vi "USRP oneTx one Rx_USRP1.vi"() -> ()   [LabVIEW 2021]
uses:
  <vilib>/addons/Modulation/Analog/controls/Complex Data Waveform.ctl
  <vilib>/measure/maspectr.llb/Power Spectrum and PSD Export Mode.ctl
  system stop.vi
  <vilib>/measure/matone.llb/Extract Single Tone Information 1 Chan (CDB).vi
  <vilib>/measure/maspectr.llb/FFT Power Spectrum and PSD for 1 Chan (CDB).vi
  <instrlib>/niUSRP/niUSRP Fetch Rx Data (CDB Cluster).vi
  <instrlib>/niUSRP/niUSRP Write Tx Data (CDB Cluster).vi
  <vilib>/addons/Modulation/niAMT.lvlib
  <vilib>/measure/NI_MAPro.lvlib
panel:
  in  "Tab Control":T1(tab)
  in  "IQ rate Tx":dbl=100000.0 format="%#_6p"
  in  "carrier frequency Tx":dbl=100000.0 format="%#_6p"
  in  "Tx Gain":dbl format="%#_6f"
  in  "Tx IP":refnum<k15>
  out "coerced IQ rate Tx":dbl=100000.0 format="%#_6p"
  out "coerced carrier frequency Tx":dbl=100000.0 format="%#_6p"
  in  "Rx IP":refnum<k15>
  in  "Rx gain":dbl format="%#_6f"
  in  "Frequency":dbl format="%#_13g"
  in  "Duration":dbl format="%#_13g"
  out "coerced IQ rate Rx":dbl=100000.0 format="%#_6p"
  out "coerced carrier frequency Rx":dbl=100000.0 format="%#_6p"
  in  "number of samples":i64=100000
  out "Waveform Graph":dbl[](graph)
  out "Boolean":bool
  out "Received Waveform Graph":cluster{"f0":dbl, "df":dbl, "magnitude":dbl[]}(graph)
  out "detected frequency":dbl format="%.2p"
  out "detected Amplitude in dBm":dbl format="%.2p"
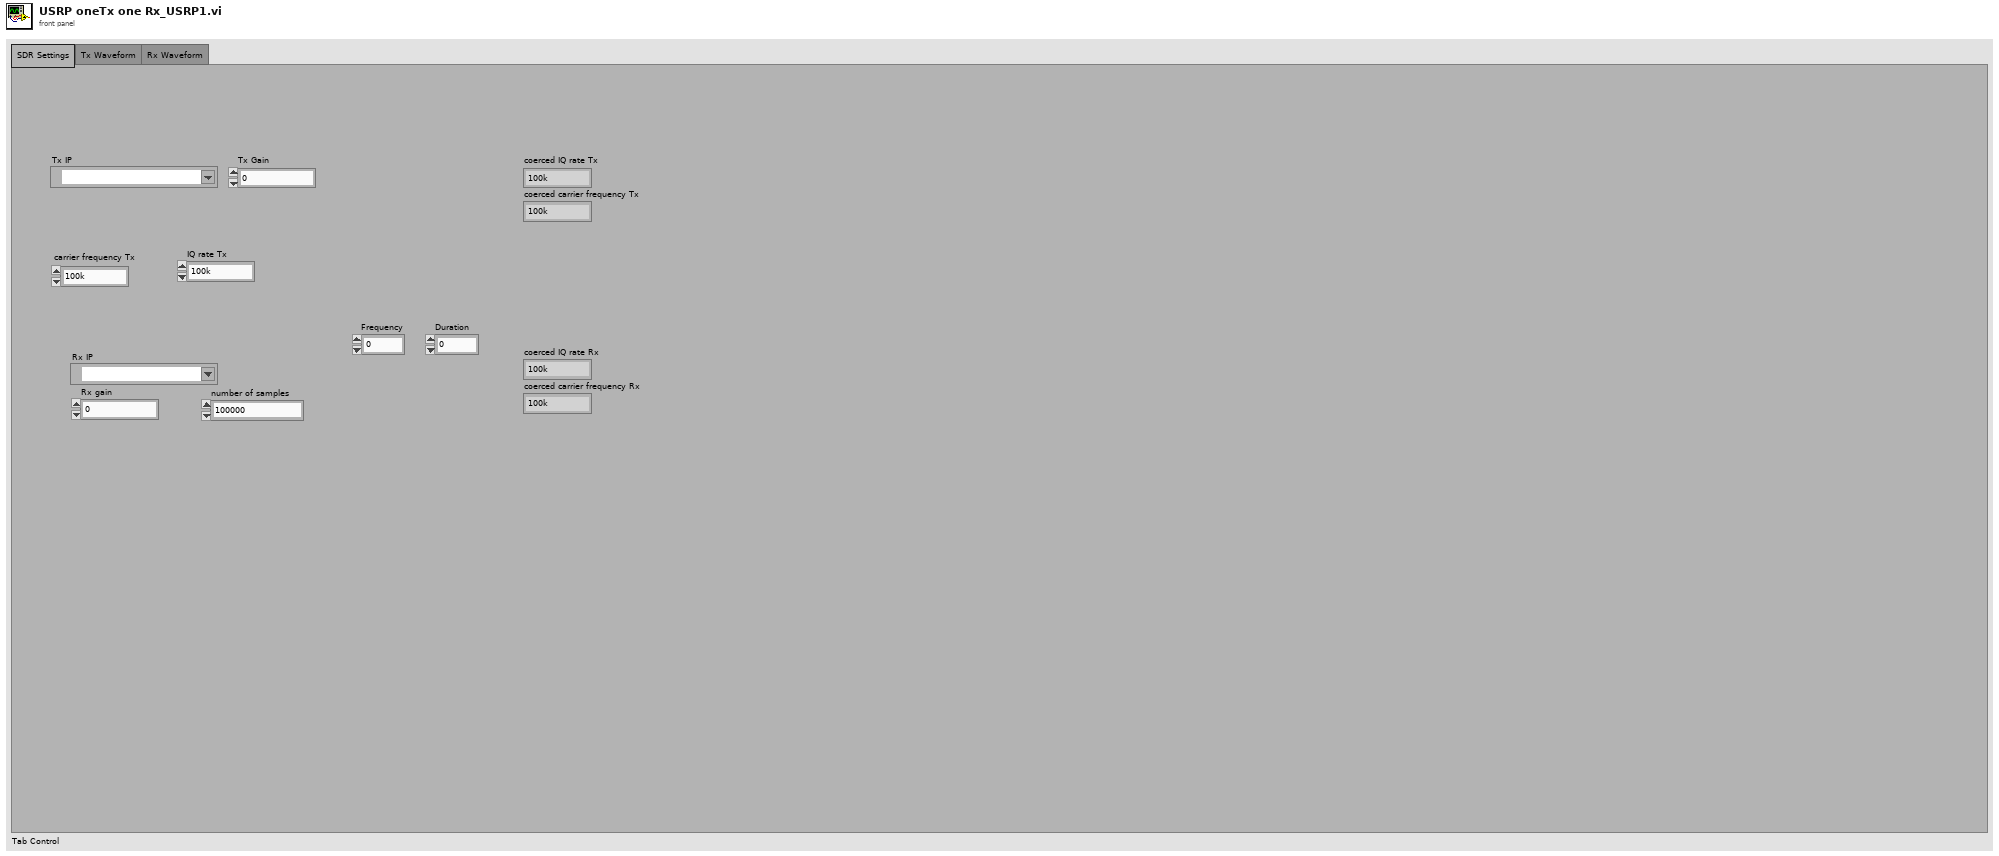
[diagram p1: front panel]
types:
  T1 = enum32{"SDR Settings", "Tx Waveform", "Rx Waveform"}
  T2 = typedef "niAMT.lvlib/Complex Data Waveform.ctl" = cluster{"t0":dbl, "dt":dbl, "Y":cdb[]}
  T3 = typedef "NI_MAPro.lvlib/Power Spectrum and PSD Export Mode.ctl" = u16
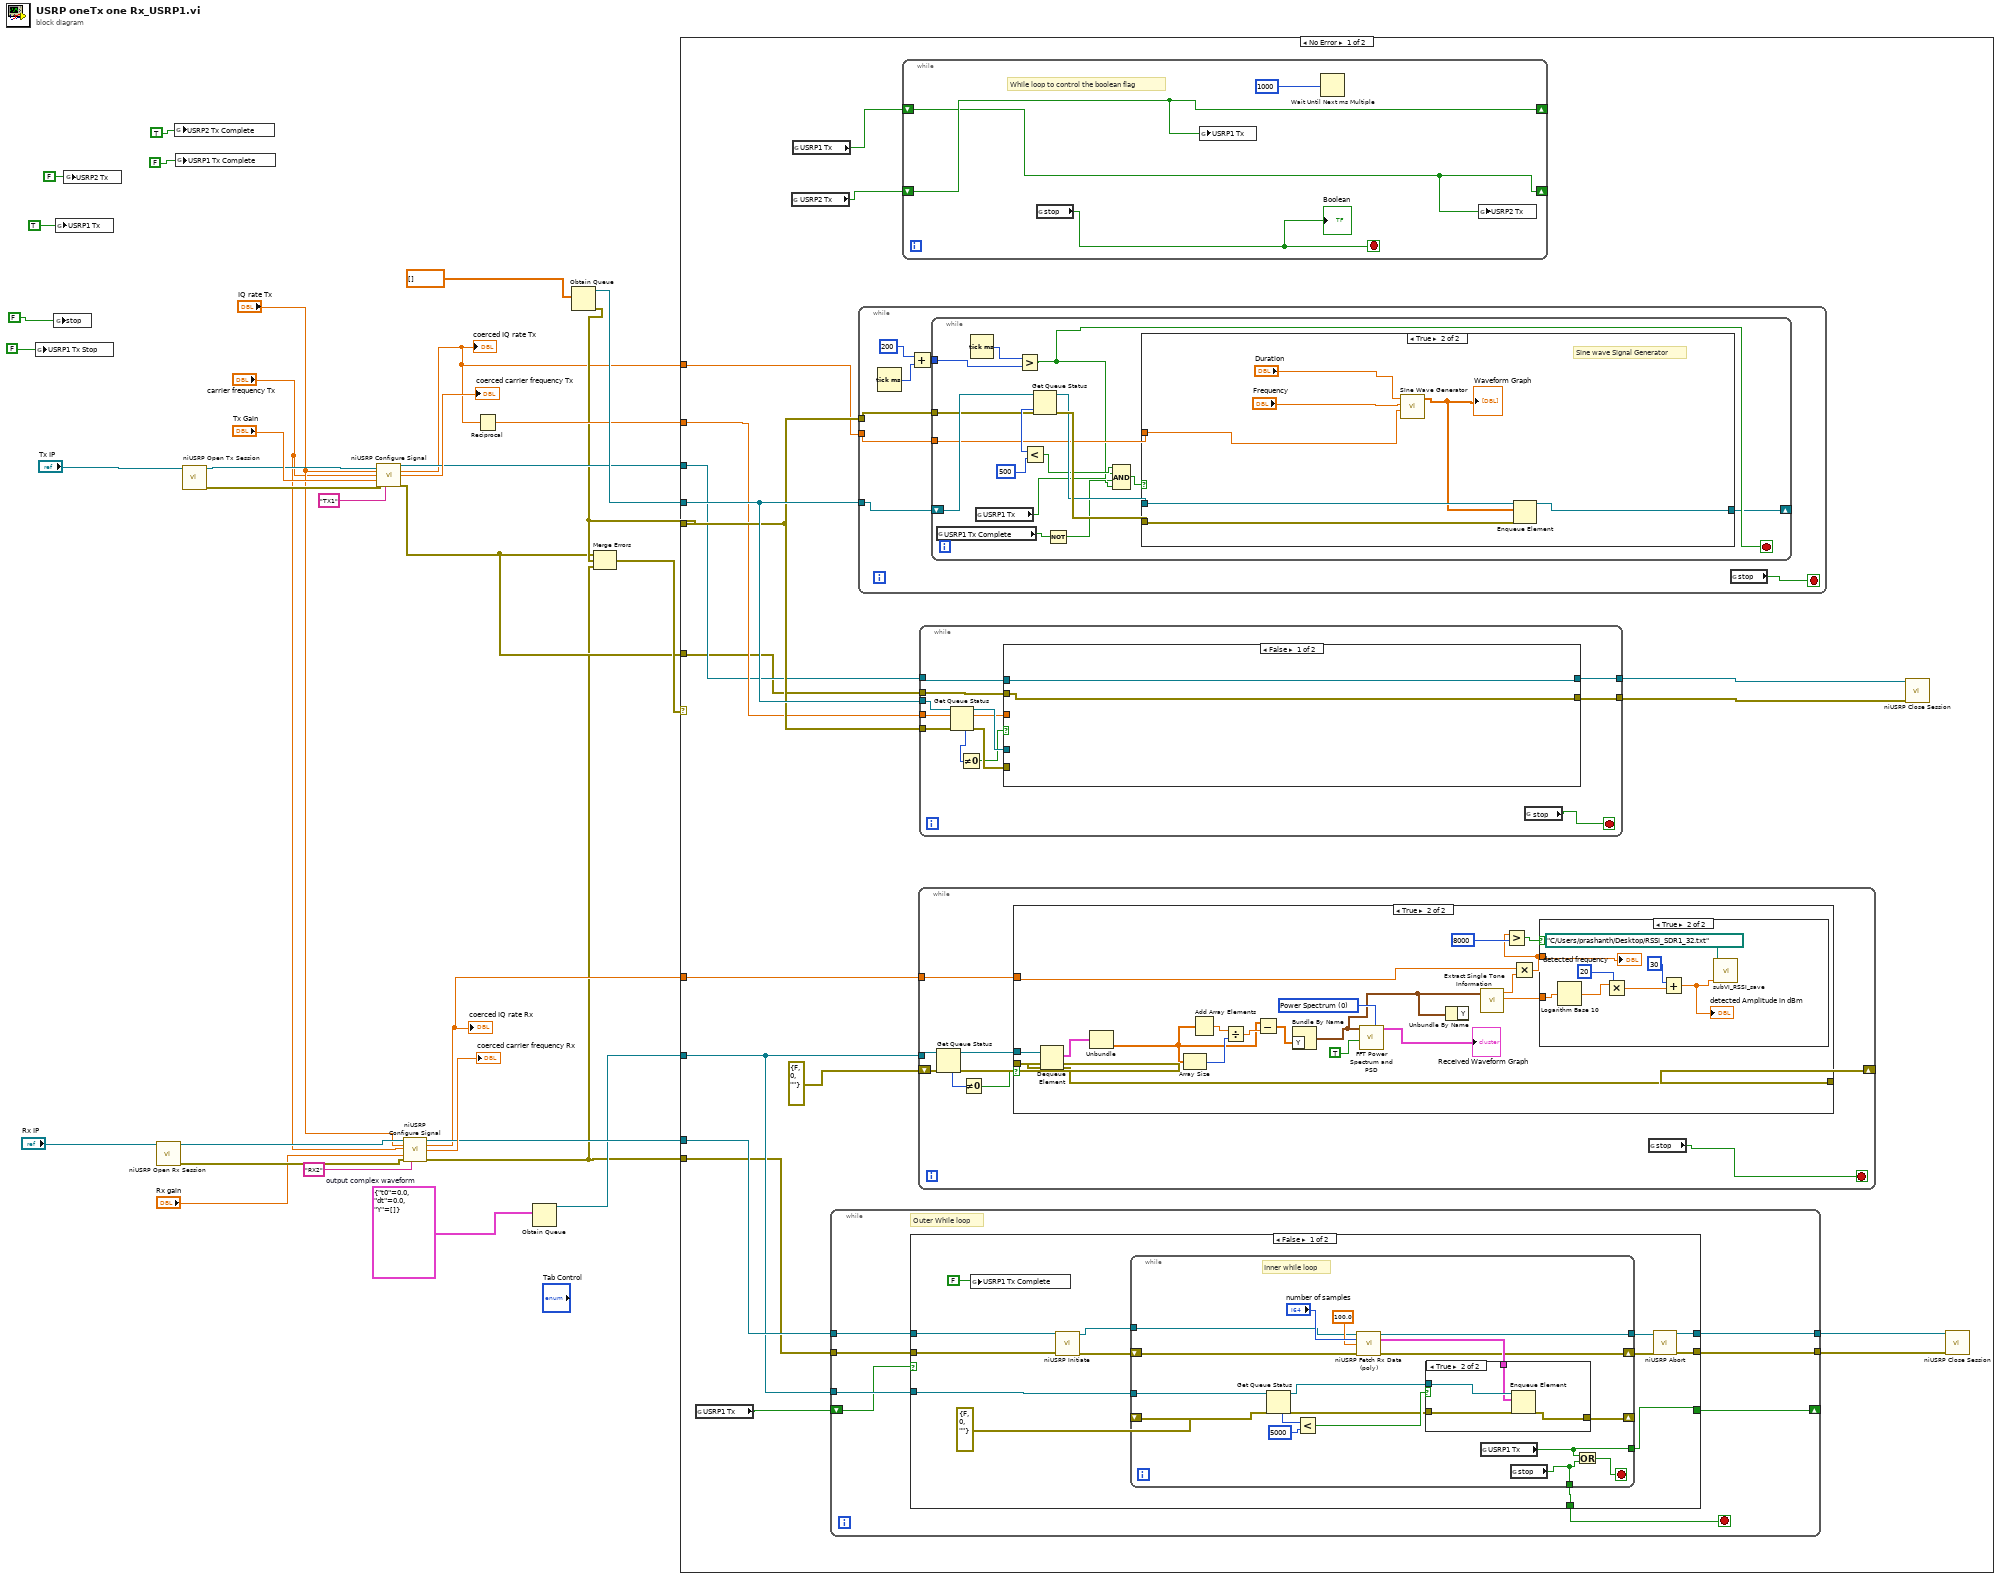
[diagram p0: block diagram]
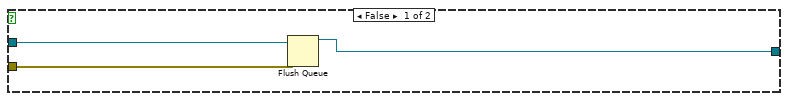
[diagram p2: hidden frame]
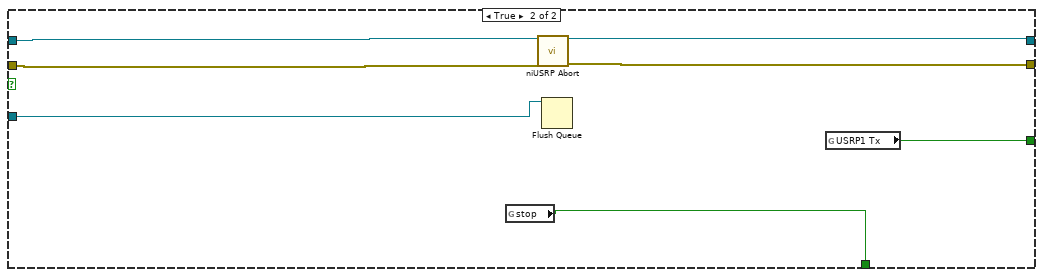
[diagram p4: hidden frame]
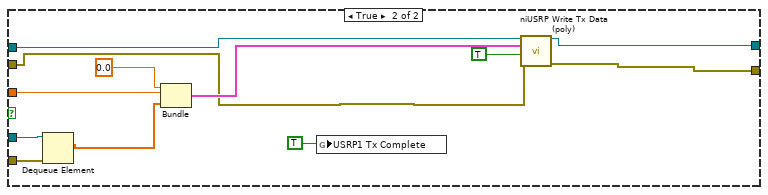
[diagram p7: hidden frame]
diagram:
  w10 = T2 {"t0"=0.0, "dt"=0.0, "Y"=[]}  # output complex waveform
  n1 = global write "system stop.vi" "USRP1 Tx Stop"(FALSE) -> ()
  n2 = global write "system stop.vi" "stop"(FALSE) -> ()
  n3 = global write "system stop.vi" "USRP1 Tx"(TRUE) -> ()
  n4 = global write "system stop.vi" "USRP2 Tx"(FALSE) -> ()
  n5 = call <instrlib>:"niUSRP Open Rx Session.vi"("device names"="Rx IP") -> ("session handle out"=w17:refnum<k15>, "error out"=w16:errorcluster)  [unwired: 13 in]
  n6 = global write "system stop.vi" "USRP2 Tx Complete"(TRUE) -> ()
  n7 = global write "system stop.vi" "USRP1 Tx Complete"(FALSE) -> ()
  n8 = call <instrlib>:"niUSRP Open Tx Session.vi"("device names"="Tx IP") -> ("session handle out"=w31:refnum<k15>, "error out"=w30:errorcluster)  [unwired: 13 in]
  n9 = call <instrlib>:"niUSRP Configure Signal.vi"("session handle"=w31, "IQ rate"="IQ rate Tx", "carrier frequency"="carrier frequency Tx", "gain"="Tx Gain", "error in (no error)"=w30, "active antenna"="TX1") -> ("session handle out"=w24:refnum<k15>, "coerced IQ rate"=w21:dbl, "coerced carrier frequency"=→"coerced carrier frequency Tx":dbl, "error out"=w20:errorcluster)  [unwired: 5 in, 1 out]
  "coerced IQ rate Tx" <- w21
  n10 = call <instrlib>:"niUSRP Configure Signal.vi"("session handle"=w17, "IQ rate"="IQ rate Tx", "carrier frequency"="carrier frequency Tx", "gain"="Rx gain", "error in (no error)"=w16, "active antenna"="RX2") -> ("session handle out"=w11:refnum<k15>, "coerced IQ rate"=w8:dbl, "coerced carrier frequency"=→"coerced carrier frequency Rx":dbl, "error out"=w6:errorcluster)  [unwired: 5 in, 1 out]
  "coerced IQ rate Rx" <- w8
  n11 = Reciprocal(x=w21) -> (1/x=w23:dbl)
  n12 = Obtain Queue(element data type=w10) -> (queue out=w9:refnum<queue>)  [unwired: 4 in, 2 out]
  n13 = Obtain Queue(element data type=dbl[] []) -> (queue out=w25:refnum<queue>, error out=w22:errorcluster)  [unwired: 4 in, 1 out]
  n14 = Merge Errors(w20, w22, w6) -> (w27:errorcluster)
  n15 = case shown="No Error" w27 {
    tunnel: w22 -> [w50 _]
    tunnel: w25 -> [w51 _]
    tunnel: w24 -> [w48 _]
    tunnel: w23 -> [w49 _]
    tunnel: w21 -> [w47 _]
    tunnel: w20 -> [w46 _]
    tunnel: w11 -> [w44 _]
    tunnel: w9 -> [w43 _]
    tunnel: w8 -> [w42 _]
    tunnel: w6 -> [w41 _]
    frame No Error {
      n16 = global read "system stop.vi" "USRP1 Tx"() -> (w36:bool)
      n17 = global read "system stop.vi" "USRP2 Tx"() -> (w34:bool)
      n18 = global read "system stop.vi" "USRP1 Tx"() -> (w35:bool)
      n19 = while {
        tunnel: w44 -> [w96]
        tunnel: w43 -> [w95]
        tunnel: w41 -> [w93]
        tunnel: [w92] -> w38
        tunnel: [w91] -> w37
        shift-right: [w89] -> _
        shift-left: w36 -> [w90]
        stop <- w94 stop-if-true
        # "Outer While loop"
        n20 = case shown="False" w90 {
          tunnel: w96 -> [w104 w137]
          tunnel: w95 -> [w109 w133]
          tunnel: [w107 w139] -> w94
          tunnel: w93 -> [w102 w135]
          tunnel: [w99 w136] -> w92
          tunnel: [w98 w134] -> w91
          tunnel: [w106 w138] -> w89
          frame False {
            n21 = global write "system stop.vi" "USRP1 Tx Complete"(FALSE) -> ()
            n22 = call <instrlib>:"niUSRP Initiate.vi"("session handle"=w104, "error in (no error)"=w102) -> ("session handle out"=w103:refnum<k15>, "error out"=w101:errorcluster)  [unwired: 12 in]
            n23 = while {
              tunnel: w109 -> [w127]
              shift-right: [w110] -> w97
              shift-left: w101 -> [w112]
              shift-right: [w126] -> _
              shift-left: errorcluster {"status"=FALSE, "code"=0, "source"=""} ("error in (no error)") -> [w125]
              tunnel: [w116] -> w107
              tunnel: [w115] -> w106
              tunnel: w103 -> [w113]
              tunnel: [w111] -> w100
              stop <- w117 stop-if-true
              # "Inner while loop"
              n24 = Get Queue Status(queue=w127, error in (no error)=w125) -> (queue out=w120:refnum<queue>, error out=w121:errorcluster, # elements in queue=w124:i32)  [unwired: 1 in, 5 out]
              n25 = Less?(x=w124, y=5000) -> (x < y?=w122:bool)
              n26 = call-poly <instrlib>:"niUSRP Fetch Rx Data (poly).vi"("session handle"=w113, "number of samples"="number of samples", "timeout"=100.0, "error in (no error)"=w112) -> ("session handle out"=w111:refnum<k15>, "data"=w118:cluster{"t0":dbl, "dt":dbl, "Y":cdb[]}, "error out"=w110:errorcluster)  [unwired: 8 in, 1 out]
              n27 = case shown="True" w122 {
                tunnel: w121 -> [w128 w132]
                tunnel: w120 -> [_ w131]
                tunnel: w118 -> [_ w130]
                tunnel: [w128 w129] -> w126
                frame False {
                }
                frame True {
                  n28 = Enqueue Element(queue=w131, element=w130, error in (no error)=w132) -> (error out=w129:errorcluster)  [unwired: 1 in, 2 out]
                }
              }
              n29 = global read "system stop.vi" "USRP1 Tx"() -> (w115:bool)
              n30 = global read "system stop.vi" "stop"() -> (w116:bool)
              n31 = Or(x=w115, y=w116) -> (x .or. y?=w117:bool)
            }
            n32 = call <instrlib>:"niUSRP Abort.vi"("session handle"=w100, "error in (no error)"=w97) -> ("session handle out"=w99:refnum<k15>, "error out"=w98:errorcluster)  [unwired: 12 in]
          }
          frame True {
            n33 = global read "system stop.vi" "stop"() -> (w139:bool)
            n34 = call <instrlib>:"niUSRP Abort.vi"("session handle"=w137, "error in (no error)"=w135) -> ("session handle out"=w136:refnum<k15>, "error out"=w134:errorcluster)  [unwired: 12 in]
            n35 = Flush Queue(queue=w133) -> ()  [unwired: 1 in, 3 out]
            n36 = global read "system stop.vi" "USRP1 Tx"() -> (w138:bool)
          }
        }
      }
      n37 = while {
        tunnel: w51 -> [w62]
        tunnel: w50 -> [w61]
        tunnel: w47 -> [w60]
        stop <- w59 stop-if-true
        n38 = Tick Count (ms)() -> (millisecond timer value=w57:u32)
        n39 = Add(x=200, y=w57) -> (x+y=w56:u32)
        n40 = while {
          tunnel: w61 -> [w73]
          tunnel: w60 -> [w72]
          tunnel: w56 -> [w67]
          shift-right: [w63] -> _
          shift-left: w62 -> [w74]
          stop <- w66 stop-if-true
          n41 = global read "system stop.vi" "USRP1 Tx Complete"() -> (w65:bool)
          n42 = Tick Count (ms)() -> (millisecond timer value=w68:u32)
          n43 = global read "system stop.vi" "USRP1 Tx"() -> (w70:bool)
          n44 = Greater?(x=w68, y=w67) -> (0:w66:bool)
          n45 = Get Queue Status(queue=w74, error in (no error)=w73) -> (queue out=w75:refnum<queue>, error out=w76:errorcluster, # elements in queue=w78:i32)  [unwired: 1 in, 5 out]
          n46 = Less?(x=w78, y=500) -> (x < y?=w71:bool)
          n47 = Not(x=w65) -> (.not. x?=w64:bool)
          n48 = Compound Arithmetic op=AND(w71, w70, w64, w66) -> (w69:bool)
          n49 = case shown="True" w69 {
            tunnel: w76 -> [w80 w88]
            tunnel: w75 -> [w81 w87]
            tunnel: w72 -> [_ w84]
            tunnel: [w79 w82] -> w63
            frame False {
              n50 = Flush Queue(queue=w81, error in (no error)=w80) -> (queue out=w79:refnum<queue>)  [unwired: 2 out]
            }
            frame True {
              # "Sine wave Signal Generator"
              n51 = call "SIne Wave Generator.vi"("Sampling rate"=w84, "Frequency"="Frequency", "Duration"="Duration") -> ("Array"=w83:dbl[])  [unwired: 7 in, 1 out]
              "Waveform Graph" <- w83
              n52 = Enqueue Element(queue=w87, element=w83, error in (no error)=w88) -> (queue out=w82:refnum<queue>)  [unwired: 1 in, 2 out]
            }
          }
        }
        n53 = global read "system stop.vi" "stop"() -> (w59:bool)
      }
      n54 = while {
        shift-right: [w54] -> _
        shift-left: w35 -> [w53]
        shift-right: [w53] -> _
        shift-left: w34 -> [w54]
        stop <- w52 stop-if-true
        # "While loop to control the boolean flag"
        n55 = global read "system stop.vi" "stop"() -> (w52:bool)
        "Boolean" <- w52
        n56 = global write "system stop.vi" "USRP1 Tx"(w54) -> ()
        n57 = Wait Until Next ms Multiple(millisecond multiple=1000) -> ()  [unwired: 1 out]
        n58 = global write "system stop.vi" "USRP2 Tx"(w53) -> ()
      }
      n59 = while {
        tunnel: w43 -> [w145]
        shift-right: [w142] -> _
        shift-left: errorcluster {"status"=FALSE, "code"=0, "source"=""} ("error in (no error)") -> [w144]
        tunnel: w42 -> [w141]
        stop <- w140 stop-if-true
        n60 = Get Queue Status(queue=w145, error in (no error)=w144) -> (queue out=w147:refnum<queue>, error out=w146:errorcluster, # elements in queue=w148:i32)  [unwired: 1 in, 5 out]
        n61 = Not Equal To 0?(x=w148) -> (x != 0?=w143:bool)
        n62 = case shown="True" w143 {
          tunnel: w147 -> [_ w168]
          tunnel: w146 -> [w149 w162]
          tunnel: [w149 w160] -> w142
          tunnel: w141 -> [_ w159]
          frame False {
          }
          frame True {
            w165 = T3 0 items=["Power Spectrum", "Power Spectral Density"] ("export mode")
            n63 = Dequeue Element(queue=w168, error in (no error)=w162) -> (element=w161:T2, error out=w160:errorcluster)  [unwired: 1 in, 2 out]
            n64 = Unbundle(w161) -> ("Y"=w151:cdb[])  [unwired: 2 out]
            n65 = Array Size(array=w151) -> (size(s)=w153:i32)
            n66 = Add Array Elements(numeric array=w151) -> (sum=w154:cdb)
            n67 = Divide(x=w154, y=w153) -> (x/y=w152:cdb)
            n68 = Subtract(x=w151, y=w152) -> (x-y=w150:cdb[])
            n69 = Bundle By Name("Y"=w150) -> (w163:waveform(cdb))  [unwired: 1 in]
            n70 = call-poly <vilib>:"FFT Power Spectrum and PSD.vi"("export mode"=w165, "dB On (F)"=TRUE, "time signal"=w163) -> ("Power Spectrum / PSD"=→"Received Waveform Graph":cluster{"f0":dbl, "df":dbl, "magnitude":dbl[]})  [unwired: 5 in, 3 out]
            n71 = Unbundle By Name(w163) -> ()  [unwired: 1 out]
            n72 = call-poly <vilib>:"Extract Single Tone Information.vi"("time signal in"=w163) -> ("detected amplitude"=w156:dbl, "detected frequency"=w164:dbl)  [unwired: 5 in, 4 out]
            n73 = Multiply(x=w159, y=w164) -> (x*y=w155:dbl)
            n74 = Greater?(x=w155, y=8000) -> (0:w158:bool)
            n75 = case shown="True" w158 {
              tunnel: w156 -> [_ w172]
              tunnel: w155 -> [_ w175]
              frame False {
              }
              frame True {
                n76 = Logarithm Base 10(1:w172) -> (0:w174:dbl)
                n77 = Multiply(x=w174, y=20) -> (x*y=w170:dbl)
                n78 = Add(x=30, y=w170) -> (x+y=w169:dbl)
                "detected Amplitude in dBm" <- w169
                n79 = call "subVI_RSSI_save.vi"("RSSI"=w169, "file path (dialog if empty)"=path "C:/Users/prashanth/Desktop/RSSI_SDR1_32.txt") -> ()  [unwired: 10 in]
                "detected frequency" <- w175
              }
            }
          }
        }
        n80 = global read "system stop.vi" "stop"() -> (w140:bool)
      }
      n81 = while {
        tunnel: w51 -> [w188]
        tunnel: w50 -> [w185]
        tunnel: w49 -> [w184]
        tunnel: w48 -> [w182]
        tunnel: w46 -> [w180]
        tunnel: [w178] -> w40
        tunnel: [w177] -> w39
        stop <- w179 stop-if-true
        n82 = Get Queue Status(queue=w188, error in (no error)=w185) -> (queue out=w187:refnum<queue>, error out=w186:errorcluster, # elements in queue=w183:i32)  [unwired: 1 in, 5 out]
        n83 = Not Equal To 0?(x=w183) -> (x != 0?=w181:bool)
        n84 = case shown="False" w181 {
          tunnel: w187 -> [_ w202]
          tunnel: w186 -> [_ w201]
          tunnel: w184 -> [_ w200]
          tunnel: w182 -> [w190 w198]
          tunnel: w180 -> [w189 w191]
          tunnel: [w190 w194] -> w178
          tunnel: [w189 w192] -> w177
          frame False {
          }
          frame True {
            n85 = Dequeue Element(queue=w202, error in (no error)=w201) -> (element=w197:dbl[])  [unwired: 1 in, 3 out]
            n86 = Bundle(0.0, w200, w197) -> (w199:cluster{dbl, dbl, dbl[]})  [unwired: 1 in]
            n87 = global write "system stop.vi" "USRP1 Tx Complete"(TRUE) -> ()
            n88 = call-poly <instrlib>:"niUSRP Write Tx Data (poly).vi"("session handle"=w198, "data"=w199, "end of data?"=TRUE, "error in (no error)"=w191) -> ("session handle out"=w194:refnum<k15>, "error out"=w192:errorcluster)  [unwired: 10 in]
          }
        }
        n89 = global read "system stop.vi" "stop"() -> (w179:bool)
      }
      n90 = call <instrlib>:"niUSRP Close Session.vi"("session handle"=w40, "error in (no error)"=w39) -> ()  [unwired: 13 in, 1 out]
      n91 = call <instrlib>:"niUSRP Close Session.vi"("session handle"=w38, "error in (no error)"=w37) -> ()  [unwired: 13 in, 1 out]
    }
    frame Error {
    }
  }
